vi "LVClasse_SurfaceFloat ctor from copy.vi"(0 "SurfaceFloat (const)":refnum<class "SurfaceFloat.lvclass">, 5 "SurfaceFloat to copy":refnum<class "SurfaceFloat.lvclass">, 11 "error in (no error)":errorcluster) -> (4 "SurfaceFloat (new)":refnum<class "SurfaceFloat.lvclass">, 6 "SurfaceFloat to copy (dup)":refnum<class "SurfaceFloat.lvclass">, 15 "error out":errorcluster)   [LabVIEW 2020, in "SurfaceFloat.lvclass"]
doc: "Surface constructor from dimensions and steps.\n\n--------------------------------------------------------------------------------\n\n<B>SurfaceIn </B> : Constant Pointer to Surface object.\n<B>SurfaceOut </B> : Constant Pointer to Surface object.\n<B>dimensions </B> : Surface dimensions (width, height).\n<B>step </B> : Physical step x and y between the surface elements (um).\n<B>ErrorIn </B> : Error\n<B>ErrorOut </B> : Error\n\n--------------------------------------------------------------------------------"
uses:
  SurfaceFloat.lvclass
  Controls/Handle creation.ctl
  SurfaceFloat.lvclass/SurfaceFloat.ctl
  LVClasse_SurfaceFloat Read SurfaceFloat.vi
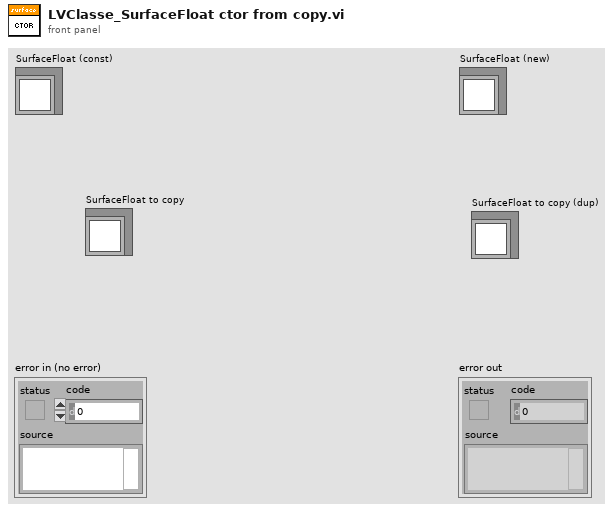
[diagram p1: front panel]
types:
  T1 = typedef "Handle creation.ctl" = enum16{"By ctor", "By write function"}
  T2 = typedef "ClassID.ctl" = i64
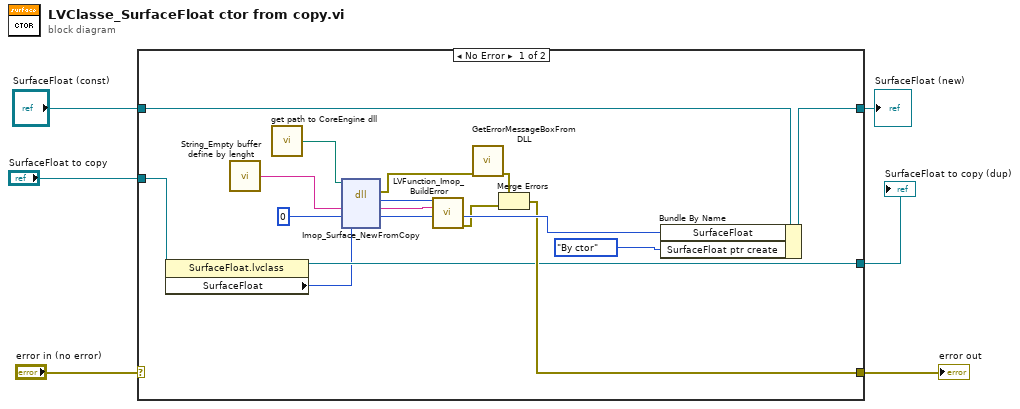
[diagram p0: block diagram]
diagram:
  n1 = case shown="No Error" "error in (no error)" {
    selector: "error in (no error)" -> [_ w25]
    tunnel: [w10 w25] -> w5
    tunnel: [w14 w24] -> w3
    tunnel: "SurfaceFloat (const)" -> [w15 w24]
    tunnel: "SurfaceFloat to copy" -> [w9 w23]
    tunnel: [w8 w23] -> w1
    frame No Error {
      n2 = property class="SurfaceFloat.lvclass"(reference=w9) -> (reference out=w8:refnum<class "SurfaceFloat.lvclass">, "SurfaceFloat"=w7:T2)  [unwired: 1 in, 1 out]
      n3 = call "String_Empty buffer define by lenght.vi"() -> ("Empty buffer"=w19:string)  [unwired: 1 in]
      n4 = call "get path to CoreEngine dll.vi"() -> ("path to wavekit library"=w18:path)  [unwired: 14 in, 1 out]
      n5 = dll-call lib="D:/soft/HASO_v3/SVN_trunk/ImOpCoreEngine4_LV2011/DLLs/c_interface_vc100.dll" fn="Imop_Surface_NewFromCopy"(path in=w18, "message"=w19, "surface"=0 ("objet"), "surface_to_copy"=w7) -> (error out=w13:errorcluster, "return type"=w22:i32, "message"=w21:string, "surface"=w20:i64)  [unwired: 3 in, 1 out]
      n6 = call "LVFunction_Imop_BuildError.vi"("code"=w22, "String to Prepend to source (\"\")"=w21) -> ("error out"=w11:errorcluster)  [unwired: 13 in]
      n7 = call "GetErrorMessageBoxFromDLL.vi"("error IN"=w13) -> ("error OUT"=w12:errorcluster)  [unwired: 10 in]
      n8 = Merge Errors(w12, w11) -> (w10:errorcluster)
      n9 = Bundle By Name(cluster=w15, "SurfaceFloat"=w20, "SurfaceFloat ptr create"=Handle_creation."By ctor" ("HasoData ptr create")) -> (w14:refnum<class "SurfaceFloat.lvclass">)
    }
    frame Error {
    }
  }
  "error out" <- w5
  "SurfaceFloat (new)" <- w3
  "SurfaceFloat to copy (dup)" <- w1
